vi "graph_error_test.vi"() -> ()   [LabVIEW 2016]
panel:
  out "Working?":bool
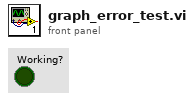
[diagram p1: front panel]
types:
  T1 = cluster{"error":cluster{"innerError":cluster{"date":string, "requestId":string}, "message":string, "code":string}}
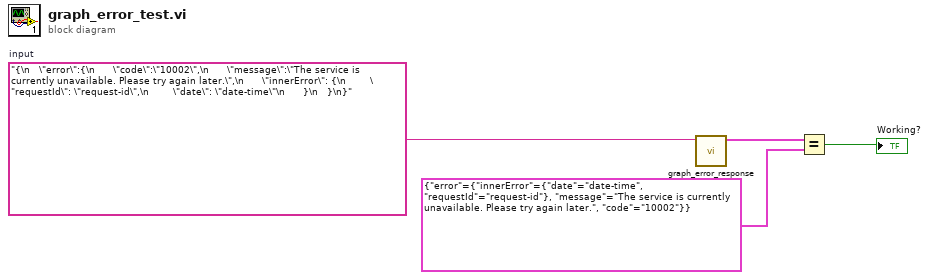
[diagram p0: block diagram]
diagram:
  w1 = "{\n   \"error\":{\n      \"code\":\"10002\",\n      \"message\":\"The service is currently unavailable. Please try again later.\",\n      \"innerError\": {\n        \"requestId\": \"request-id\",\n        \"date\": \"date-time\"\n      }\n   }\n}"  # input
  n1 = call "graph_error_response.vi"("Error Response"=w1) -> ("data"=w3:T1)  [unwired: 9 in, 1 out]
  n2 = Equal?(x=w3, y=T1 {"error"={"innerError"={"date"="date-time", "requestId"="request-id"}, "message"="The service is currently unavailable. Please try again later.", "code"="10002"}} ("data")) -> (x = y?=→"Working?":bool)
